vi "svfa_Scale FFT Array for RMS.vi"(7 "leave DC bin unscaled (T)":bool=TRUE, 10 "f0":dbl format="%.2f", 11 "FFT{X} [EU]":cdb[](array[numeric]) format="%.2f") -> (3 "FFT {X} [rms]":cdb[](array[numeric]) format="%.2f")   [LabVIEW 2017]
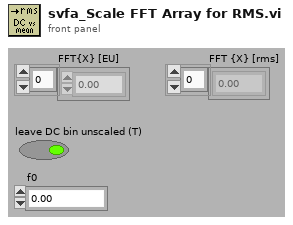
[diagram p1: front panel]
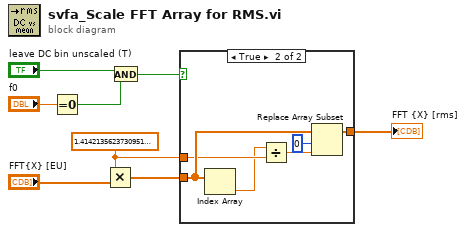
[diagram p0: block diagram]
diagram:
  w7 = cdb 1.4142135623730951+0.0i ("sqrt(x)")
  n1 = Equal To 0?(x="f0") -> (x = 0?=w3:bool)
  n2 = Multiply(x=w7, y="FFT{X} [EU]") -> (x*y=w2:cdb[])
  n3 = And(x="leave DC bin unscaled (T)", y=w3) -> (x .and. y?=w5:bool)
  n4 = case shown="True" w5 {
    tunnel: w2 -> [w9 w13]
    tunnel: w7 -> [_ w12]
    tunnel: [w9 w10] -> w1
    frame False {
    }
    frame True {
      n5 = Index Array(array=w13) -> (element=w11:cdb)  [unwired: 1 in]
      n6 = Divide(x=w11, y=w12) -> (x/y=w14:cdb)
      n7 = Replace Array Subset(array=w13, new element=w14, index=0 ("Index")) -> (w10:cdb[])
    }
  }
  "FFT {X} [rms]" <- w1
